vi "ge_CfgGroup.vi"(6 "Group Specific Info":T5={"Rate Class"=enum."Low Speed", "Chassis Name"="cDAQ9188-1630874-007"}, 7 "Mode":enum16{"Cfg", "Run"}(ring), 8 "error in":errorcluster, 11 "ChanGrp.lvclass":refnum<class "ChanGrp.lvclass">) -> (0 "error out":errorcluster, 2 "Canceled?":bool, 3 "ChanGrp.lvclass":refnum<class "ChanGrp.lvclass">)   [LabVIEW 2018]
uses:
  Custom Ctls Table/ge_PullDown.ctl
  Custom Buttons/Reset_Blue.ctl
  Classes/Cfg Grandmaster/Class Chan Group/ChanGrp.lvclass
  Custom Ctls Table/ge_CellInt.ctl
  Custom Ctls Table/ge_GrpSpecificInfo.ctl
  Common/Controls/TE_Designator.ctl
  Custom Ctls Table/ge_CellString.ctl
  Custom Ctls Table/ge_CellHiLite.ctl
  Custom Buttons/Open_BlueSmall.ctl
  Custom Buttons/Save_BlueSmall.ctl
  <vilib>/event_ctls.llb/eventvkey.ctl
  Custom Ctls Table/ge_TableCmnds.ctl
  Custom Ctls Table/ge_CellContents.ctl
  <vilib>/Utility/miscctls.llb/LVPoint32TypeDef.ctl
  <vilib>/Utility/inputDevices.llb/mouseAcquire.vi
  <vilib>/Utility/inputDevices.llb/closeMouse.vi
panel:
  in  "Save Channel List":T1
  in  "Load Descriptions":T2
  in  "Cal2":bool
  in  "Bool1":bool
  in  "CellHiLite":T3
  in  "CellString":T4=" Quarter Bridge I"
  in  "Cal1":bool
  in  "Cal0":bool
  in  "Dbl6":dbl
  in  "Dbl5":dbl=1000.0
  in  "Dbl4":dbl=1000.0
  in  "Dbl3":dbl=1000.0
  in  "Dbl2":dbl
  in  "Dbl1":dbl=1.0
  in  "Ring3":u16(ring)=10050 items=["RMS"=1, "Peak"=0, ""=65535]
  in  "CellInt":T7
  in  "CellDbl":dbl
  in  "Bool0":bool
  in  "Int0":i32
  in  "Str0":string="V"
  in  "Dbl0":dbl=25.0 format="%#.6g"
  in  "Cancel":bool
  in  "Reset":T8
  in  "Ring2":u16(ring)=10200 items=["Full Bridge I"=10183, "Full Bridge II"=10184, "Full Bridge III"=10185, "Half Bridge I"=10188, "Half Bridge II"=10189, "Quarter Bridge I"=10271, "Quarter Bridge II"=10272, ""=65535]
  in  "Ring1":u16(ring)=10086 items=["10 V"=10000, "5 V"=5000, "3.3 V"=3300, "2.5 V"=2500, ""=65535]
  in  "Ring0":u16(ring)=10144 items=["High Res"=0, ""=65535]
  in  "Pull Down":T9=65535 items=["Quarter Bridge II"=10272, "Quarter Bridge I"=10271, "Half Bridge II"=10189, "Half Bridge I"=10188, "Full Bridge III"=10185, "Full Bridge II"=10184, "Full Bridge I"=10183, ""=65535]
  in  "Apply":bool
  in  "Chan Table":i32[](listbox)
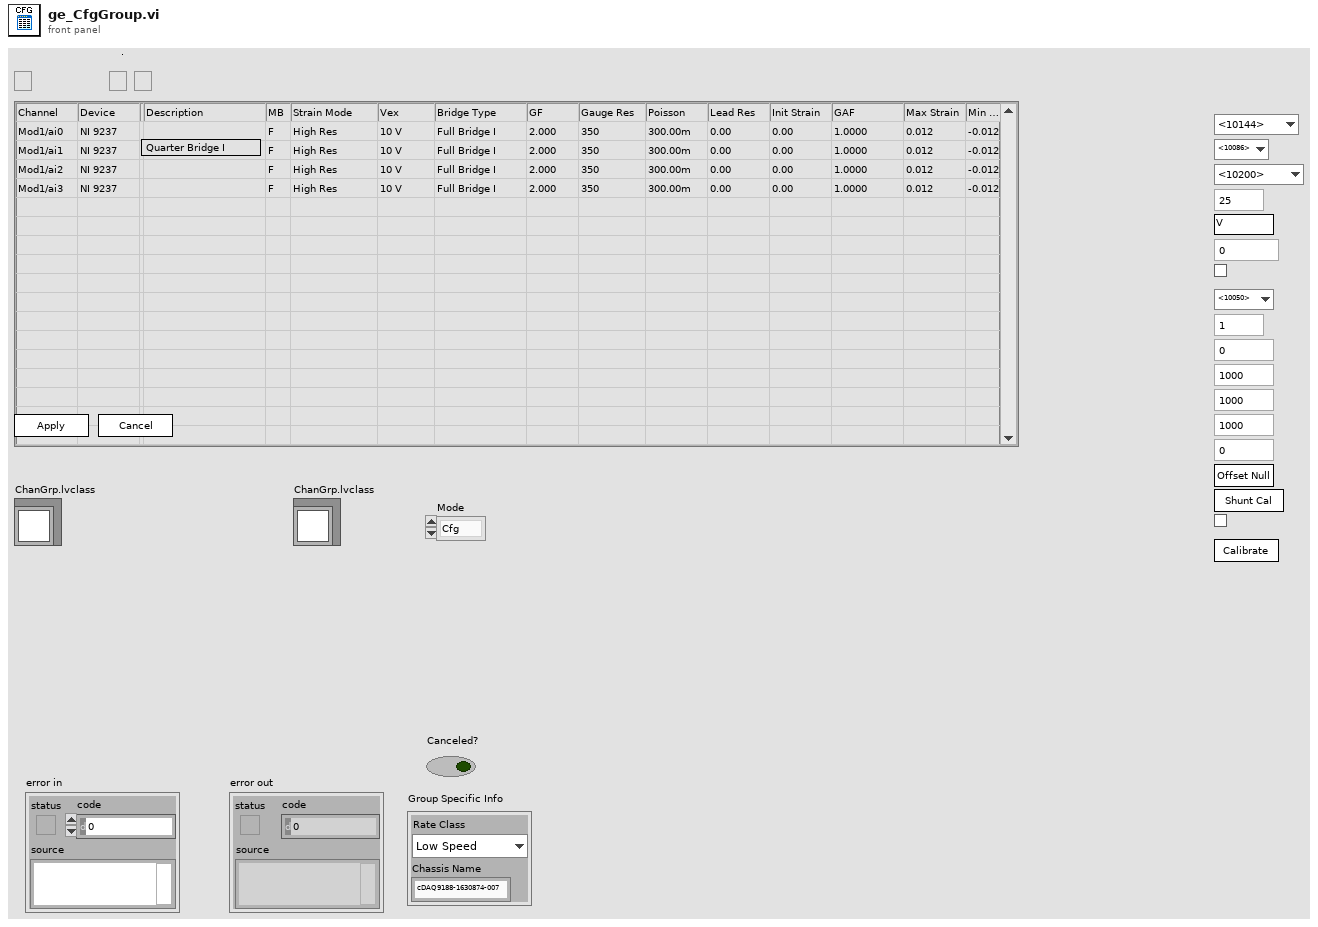
[diagram p1: front panel]
types:
  T1 = typedef "Save_BlueSmall.ctl" = bool
  T2 = typedef "Open_BlueSmall.ctl" = bool
  T3 = typedef "ge_CellHiLite.ctl" = bool
  T4 = typedef "ge_CellString.ctl" = string
  T5 = typedef "ge_GrpSpecificInfo.ctl" = cluster{"Rate Class":T6, "Chassis Name":string}
  T6 = typedef "TE_Designator.ctl" = enum16{"High Speed", "Low Speed"}
  T7 = typedef "ge_CellInt.ctl" = i32
  T8 = typedef "Reset_Blue.ctl" = bool
  T9 = typedef "ge_PullDown.ctl" = u16
  T10 = typedef "eventvkey.ctl" = enum16{"ASCII", "Enter", "Return", "Shift", "Ctrl", "Alt", "Cmd", "Opt", "Caps", "NumLock", "Clear", "Break", "Up", "Down", "Left", "Right", "Insert", "Delete", "Home", "End", "PageUp", "PageDown", "Escape", "Help", "Pause", "ScrollLock", "F1", "F2", "F3", "F4", "F5", "F6", "F7", "F8", "F9", "F10", "F11", "F12", "F13", "F14", "F15", "F16", "F17", "F18", "F19", "F20", "F21", "F22", "F23", "F24", "Play", "VolumeUp", "VolumeDown", "Mute", "Two Byte Char"}
  T11 = typedef "ge_TableCmnds.ctl" = enum16{"Initialize", "Hide Cell Ctrls", "Position Ctrls", "Load Table", "Reset Table", "Clear Selections", "Ungchd Enter?", "Cell ValChng", "Click Ring", "Edit Cell", "Dismiss Menu", "Glbl Apply", "Calibrate", "Apply Settings", "Cell Key", "SaveChanList", "LoadChanDesc", "Shutdown"}
  T12 = enum32{"Invalid", "Standard", "Closed", "Hidden", "Minimized", "Maximized"}
  T13 = cluster{"This VI":refnum<vi>, "Group Specific Info":T5}
  T14 = typedef "ge_CellContents.ctl" = cluster{"Cell Contents":cluster{"Cell Text":string, "Cell BG Color":u32}, "Coords":T15}
  T15 = typedef "LVPoint32TypeDef.ctl" = cluster{"Horizontal":i32, "Vertical":i32}
  T16 = cluster{"Horizontal":i32, "Vertical":i32, "Scrolling":i32}
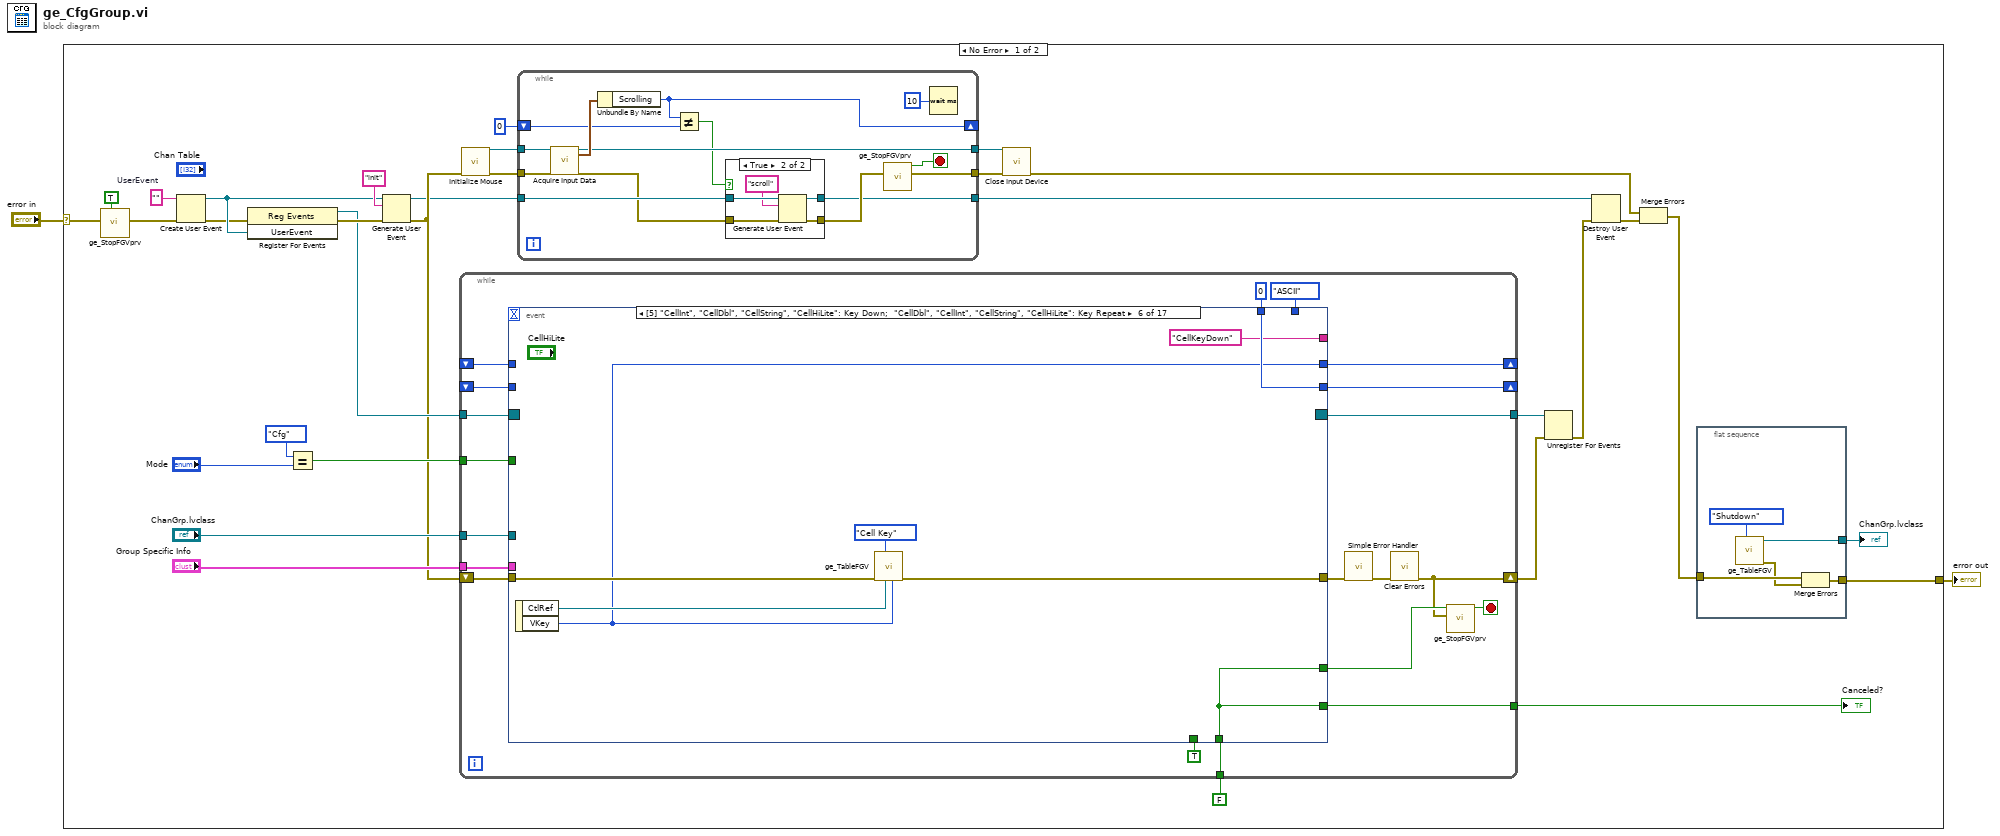
[diagram p0: block diagram]
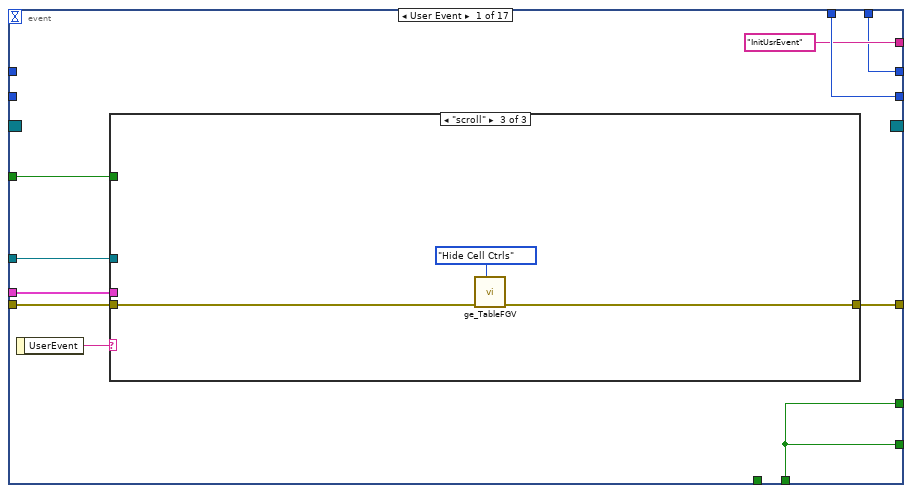
[diagram p3: hidden frame]
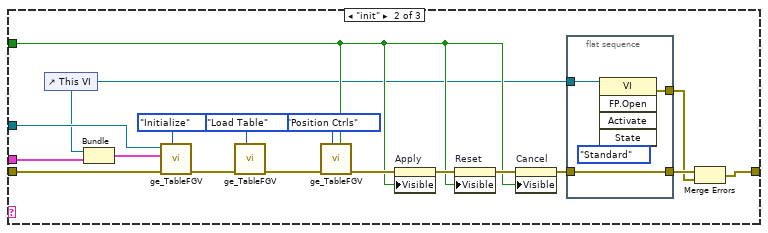
[diagram p5: hidden frame]
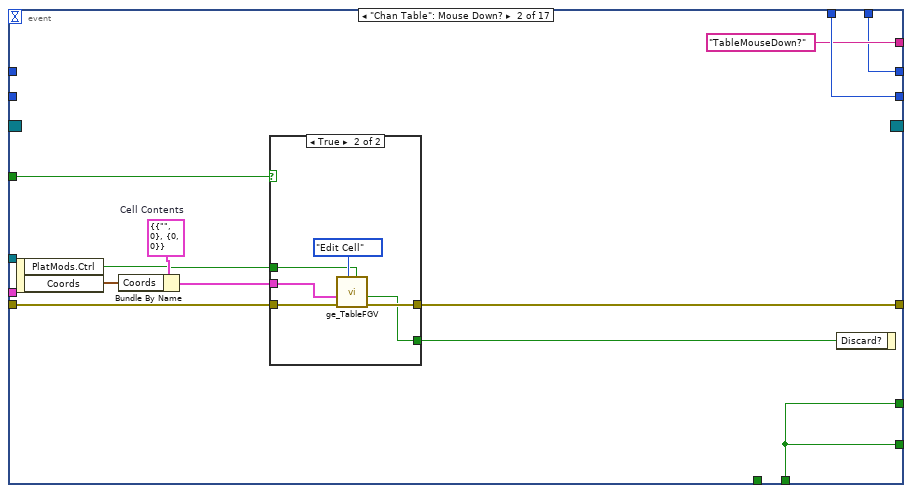
[diagram p6: hidden frame]
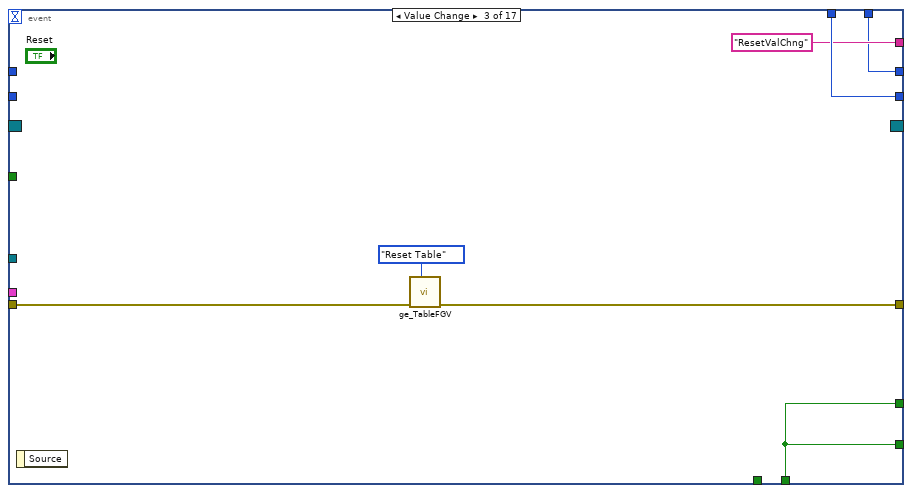
[diagram p8: hidden frame]
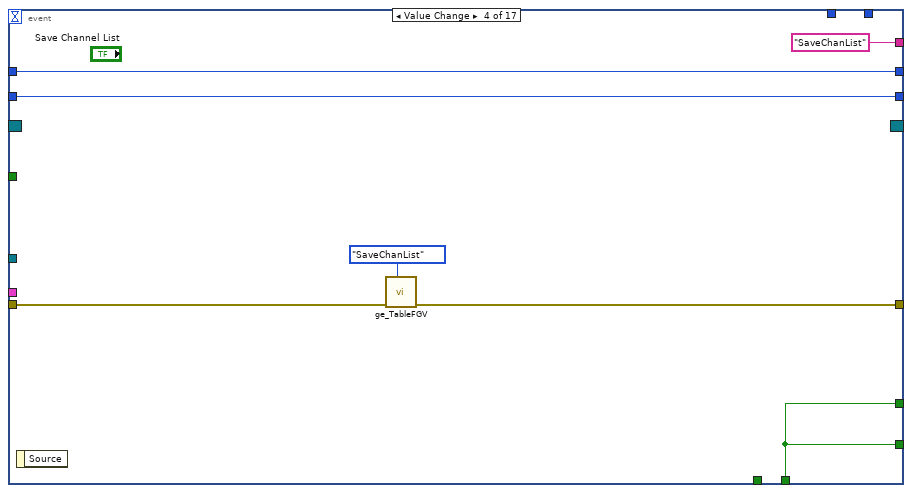
[diagram p9: hidden frame]
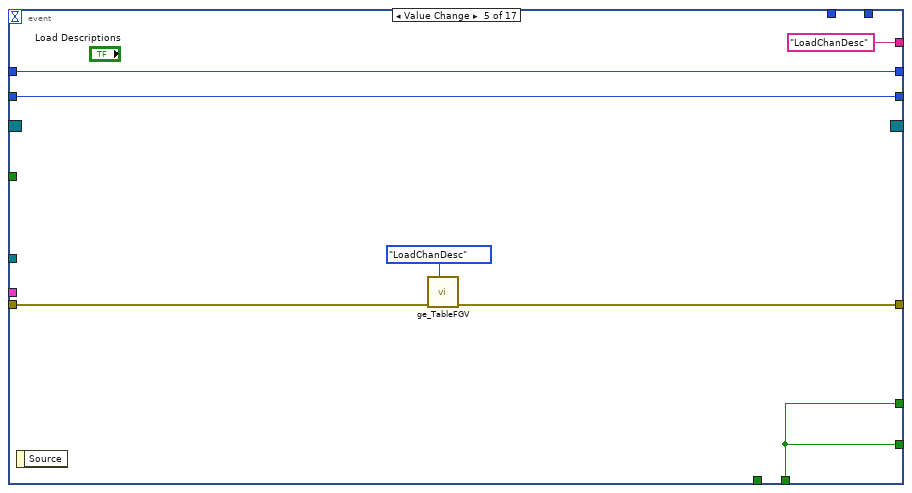
[diagram p10: hidden frame]
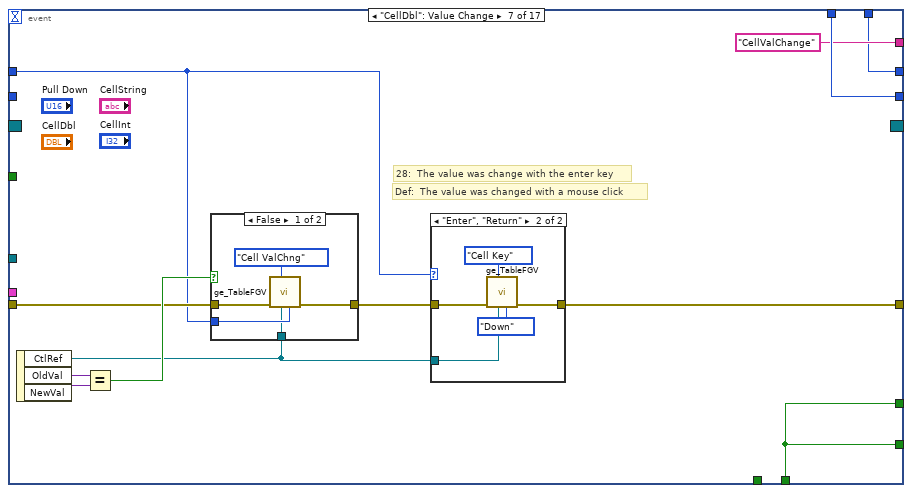
[diagram p11: hidden frame]
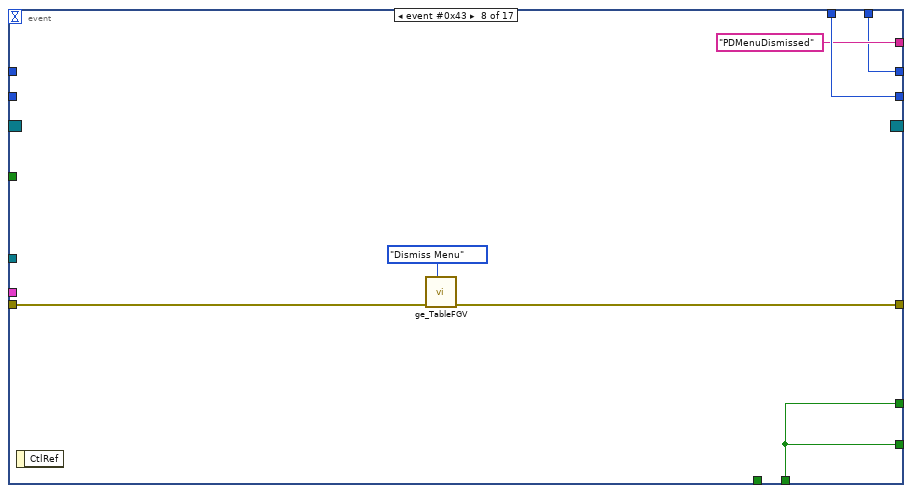
[diagram p14: hidden frame]
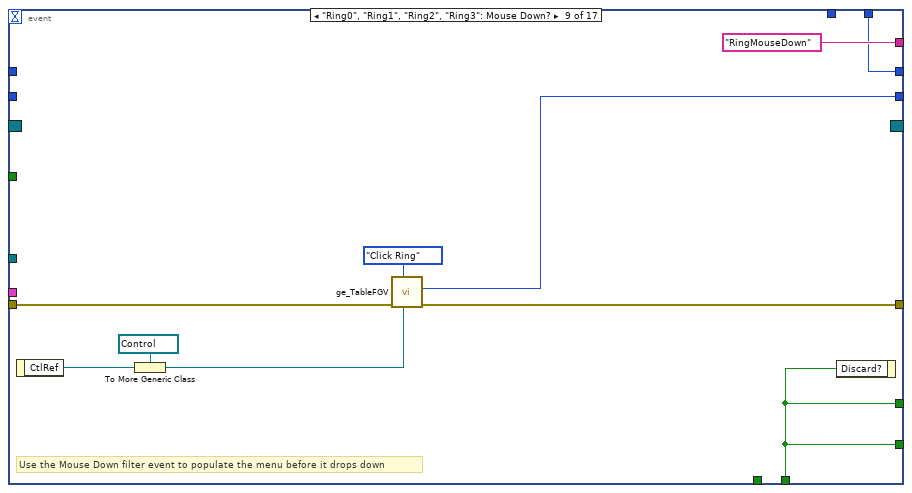
[diagram p15: hidden frame]
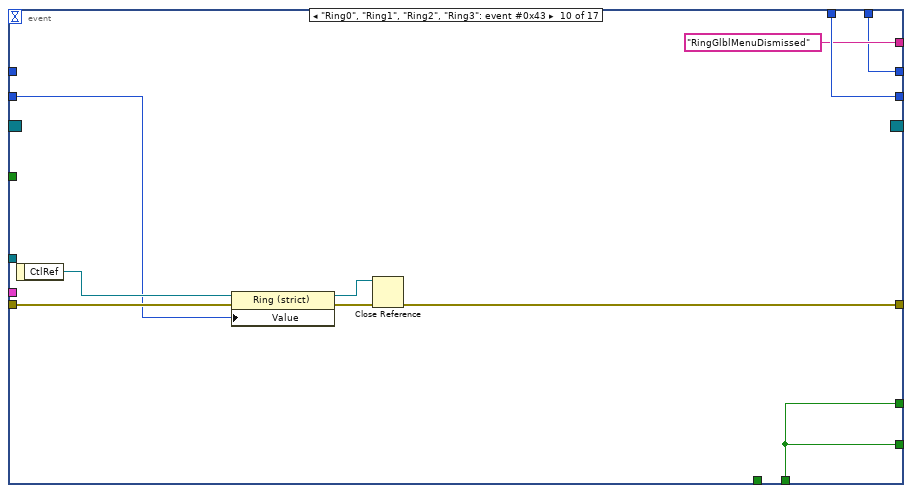
[diagram p16: hidden frame]
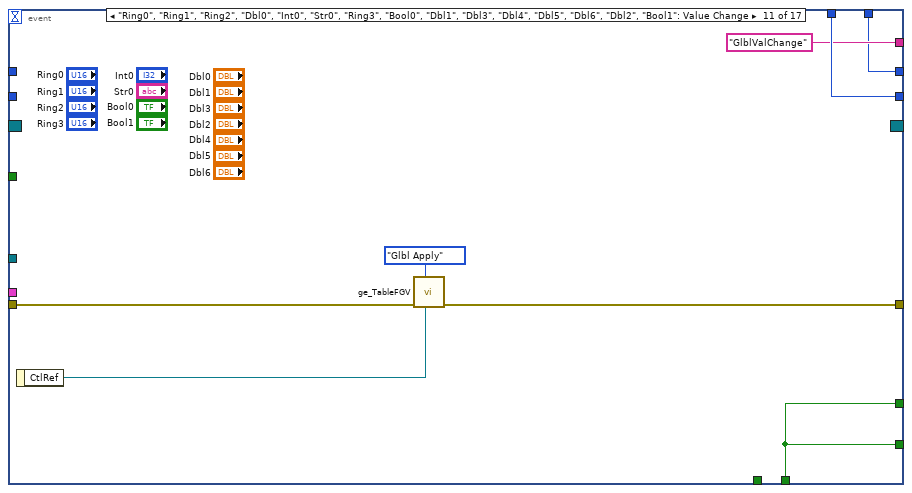
[diagram p17: hidden frame]
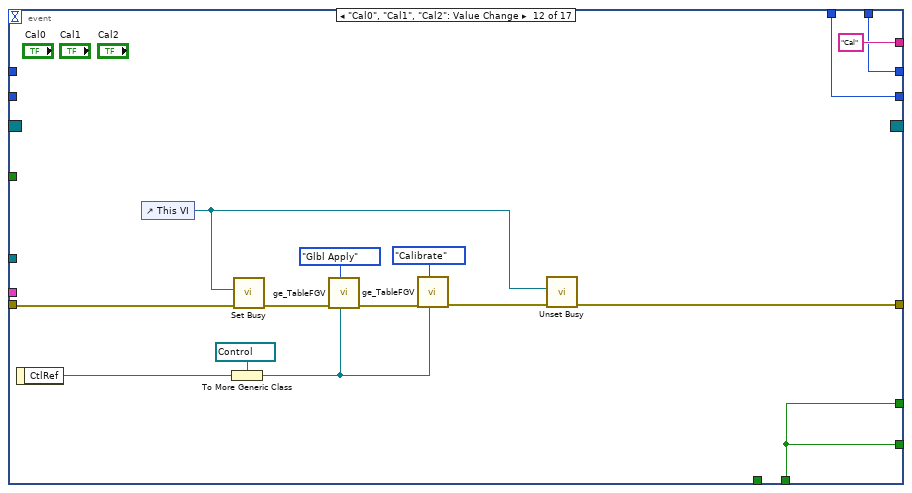
[diagram p18: hidden frame]
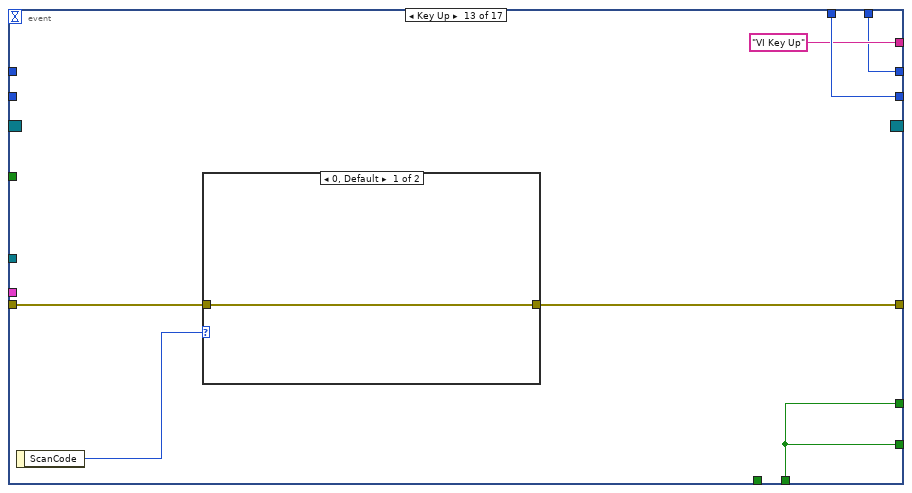
[diagram p19: hidden frame]
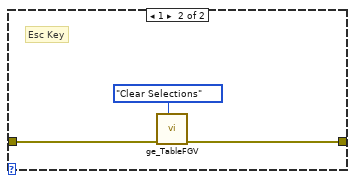
[diagram p20: hidden frame]
diagram:
  n1 = case shown="No Error" "error in" {
    selector: "error in" -> [w7 w284]
    tunnel: [w34 w284] -> w1
    frame No Error {
      w31 = ""  # UserEvent
      n2 = call "ge_StopFGVprv.vi"("Reset (F)"=TRUE, "error in"=w7) -> ("error out"=w6:errorcluster)  [unwired: 8 in, 1 out]
      n3 = Create User Event(user event datatype=w31, error in=w6) -> (user event=w29:refnum<user-event>, error out=w28:errorcluster)
      n4 = register-events(error in=w28, w29) -> (reference out=w27:refnum<event-registration>, error out=w30:errorcluster)  [unwired: 1 in]
      n5 = Equal?(x=enum16{"Cfg", "Run"}."Cfg", y="Mode") -> (x = y?=w19:bool)
      n6 = Generate User Event(user event=w29, event data cluster="init" ("event data"), error in=w30) -> (user event out=w4:refnum<user-event>, error out=w13:errorcluster)  [unwired: 1 in]
      n7 = while {
        shift-right: [w56] -> w24
        shift-left: w13 -> [w75]
        tunnel: w19 -> [w74]
        tunnel: [w72] -> w22
        tunnel: FALSE ("Apply") -> [w67]
        tunnel: "ChanGrp.lvclass" -> [w71]
        tunnel: w27 -> [w70]
        tunnel: [w69] -> w25
        shift-right: [w68] -> _
        shift-left: _ -> [w66]
        tunnel: "Group Specific Info" -> [w65]
        shift-right: [w62] -> _
        shift-left: _ -> [w61]
        stop <- w58 stop-if-true
        n8 = event shown="[5] \"CellInt\", \"CellDbl\", \"CellString\", \"CellHiLite\": Key Down;  \"CellDbl\", \"CellInt\", \"CellString\", \"CellHiLite\": Key Repeat" {
          selector: w70 -> [_ _ _ _ _ _ _ _ _ _ _ _ _ _ _ _ _]
          dyn-events: [_ _ _ _ _ _ _ _ _ _ _ _ _ _ _ _ _] -> w69
          timeout: _ -> [_ _ _ _ _ _ _ _ _ _ _ _ _ _ _ _ _]
          tunnel: [w84 w121 w135 w142 w149 w160 w172 w188 w192 w207 w219 w234 w239 w252 w265 w272 w277] -> w57
          tunnel: [w77 w123 w137 w139 w146 w158 w171 w190 w198 w208 w217 w226 w241 w250 w267 w273 w278] -> w64
          tunnel: w75 -> [w85 w122 w138 w140 w147 w159 w166 w189 w200 w210 w216 w229 w240 w253 w268 w273 w278]
          tunnel: w74 -> [w81 w115 _ _ _ _ _ _ _ _ _ _ _ _ _ _ _]
          tunnel: TRUE -> [_ _ _ _ _ _ _ _ _ _ _ _ _ _ w265 w272 w277]
          tunnel: [w84 w121 w135 w142 w149 w160 w172 w188 w192 w207 w219 w234 w239 w252 w264 w272 w277] -> w72
          tunnel: w71 -> [w83 _ _ _ _ _ _ _ _ _ _ _ _ _ _ _ _]
          tunnel: [w78 w112 w132 w144 w152 w153 w162 w185 w193 w204 w212 w220 w235 w246 w261 w269 w274] -> w68
          tunnel: w67 -> [w84 w121 w135 w142 w149 w160 w172 w188 w192 w207 w219 w234 w239 w252 w264 _ _]
          tunnel: w66 -> [_ _ _ w144 w152 _ w164 _ _ _ _ _ _ _ _ _ _]
          tunnel: w65 -> [w82 _ _ _ _ _ _ _ _ _ _ _ _ _ _ _ _]
          tunnel: [w80 w114 w134 w143 w151 w157 w165 w187 w199 w206 w214 w230 w237 w248 w263 w271 w276] -> w62
          tunnel: w61 -> [_ _ _ w143 w151 _ _ _ _ w202 _ _ _ _ _ _ _]
          tunnel: u16 0 ("RingVal") -> [w80 w114 w134 _ _ w157 w165 w187 _ w206 w214 w230 w237 w248 w263 w271 w276]
          tunnel: ["InitUsrEvent" "TableMouseDown?" "ResetValChng" "SaveChanList" "LoadChanDesc" "CellKeyDown" "CellValChange" "PDMenuDismissed" "RingMouseDown" "RingGlblMenuDismissed" "GlblValChange" "Cal" "VI Key Up" "PaneMouseDn" "ApplyValChng" "CancelValChng" "PanelClose?"] -> _
          tunnel: eventvkey."ASCII" ("VKey") -> [w78 w112 w132 _ _ _ w162 w185 w193 w204 w212 w220 w235 w246 w261 w269 w274]
          event User Event {
            n9 = event-data() -> ("UserEvent"=w76:string)  [unwired: 1 in]
            n10 = case shown="\"scroll\"" w76 {
              tunnel: w85 -> [w86 w103 w110]
              tunnel: w83 -> [_ w102 _]
              tunnel: w82 -> [_ w94 _]
              tunnel: w81 -> [_ w92 _]
              tunnel: [w86 w87 w109] -> w77
              frame Default {
              }
              frame "init" {
                n11 = control-ref of="This VI"() -> (w91:refnum<vi>)
                n12 = Bundle("This VI"=w91, "Group Specific Info"=w94) -> (w93:T13)  [unwired: 1 in]
                n13 = call "ge_TableFGV.vi"("ge_TableCmnds"=ge_TableCmnds."Initialize" ("ge_VoltTableCmnds"), "error in"=w103, "Specific Info"=w93, "ChanGrp.lvclass"=w102) -> ("error out"=w98:errorcluster)  [unwired: 4 in, 3 out]
                n14 = call "ge_TableFGV.vi"("ge_TableCmnds"=ge_TableCmnds."Load Table" ("ge_VoltTableCmnds"), "error in"=w98) -> ("error out"=w96:errorcluster)  [unwired: 6 in, 3 out]
                n15 = call "ge_TableFGV.vi"("Mod"=w92, "ge_TableCmnds"=ge_TableCmnds."Position Ctrls" ("ge_VoltTableCmnds"), "error in"=w96) -> ("error out"=w95:errorcluster)  [unwired: 5 in, 3 out]
                n16 = property on="Apply" class="Bool"(error in=w95, "Visible"=w92) -> (error out=w101:errorcluster)  [unwired: 1 in, 1 out]
                n17 = property on="Reset" class="Bool"(error in=w101, "Visible"=w92) -> (error out=w100:errorcluster)  [unwired: 1 in, 1 out]
                n18 = property on="Cancel" class="Bool"(error in=w100, "Visible"=w92) -> (error out=w90:errorcluster)  [unwired: 1 in, 1 out]
                n19 = flat-sequence {
                  tunnel: [w108] -> w88
                  tunnel: w91 -> [w106]
                  tunnel: w90 -> [w105]
                  tunnel: [w105] -> w89
                  frame #0 {
                    n20 = invoke class="VI" method="FP.Open"(reference=w106, "State"=T12."Standard") -> (error out=w108:errorcluster)  [unwired: 3 in, 4 out]
                  }
                }
                n21 = Merge Errors(w89, w88) -> (w87:errorcluster)
              }
              frame "scroll" {
                n22 = call "ge_TableFGV.vi"("ge_TableCmnds"=ge_TableCmnds."Hide Cell Ctrls" ("ge_VoltTableCmnds"), "error in"=w110) -> ("error out"=w109:errorcluster)  [unwired: 6 in, 3 out]
              }
            }
          }
          event "Chan Table": Mouse Down? {
            w120 = T14 {"Cell Contents"={"Cell Text"="", "Cell BG Color"=0}, "Coords"={"Horizontal"=0, "Vertical"=0}}  # Cell Contents
            n23 = event-data() -> ("PlatMods.Ctrl"=w116:bool, "Coords"=w119:T15)  [unwired: 1 in]
            n24 = Bundle By Name(cluster=w120, "Coords"=w119) -> (w118:T14)
            n25 = case shown="True" w115 {
              selector: w115 -> [w124 _]
              tunnel: [w125 w131] -> w123
              tunnel: w122 -> [w125 w130]
              tunnel: w118 -> [_ w128]
              tunnel: [w124 w126] -> w117
              tunnel: w116 -> [_ w127]
              frame False {
              }
              frame True {
                n26 = call "ge_TableFGV.vi"("Mod"=w127, "ge_TableCmnds"=ge_TableCmnds."Edit Cell" ("ge_VoltTableCmnds"), "error in"=w130, "Cell Contents"=w128) -> ("error out"=w131:errorcluster, "Discard?"=w126:bool)  [unwired: 4 in, 2 out]
              }
            }
            n27 = event-data("Discard?"=w117) -> ()  [unwired: 1 in, 1 out]
          }
          event Value Change {
            n28 = event-data() -> ()  [unwired: 1 in, 1 out]
            n29 = call "ge_TableFGV.vi"("ge_TableCmnds"=ge_TableCmnds."Reset Table" ("ge_VoltTableCmnds"), "error in"=w138) -> ("error out"=w137:errorcluster)  [unwired: 6 in, 3 out]
          }
          event Value Change {
            n30 = event-data() -> ()  [unwired: 1 in, 1 out]
            n31 = call "ge_TableFGV.vi"("ge_TableCmnds"=ge_TableCmnds."SaveChanList" ("ge_VoltTableCmnds"), "error in"=w140) -> ("error out"=w139:errorcluster)  [unwired: 6 in, 3 out]
          }
          event Value Change {
            n32 = event-data() -> ()  [unwired: 1 in, 1 out]
            n33 = call "ge_TableFGV.vi"("ge_TableCmnds"=ge_TableCmnds."LoadChanDesc" ("ge_VoltTableCmnds"), "error in"=w147) -> ("error out"=w146:errorcluster)  [unwired: 6 in, 3 out]
          }
          event "CellDbl": Key Down; "CellDbl": Key Repeat {
            n34 = event-data() -> ("CtlRef"=w155:refnum<vi>, "VKey"=w153:T10)  [unwired: 1 in]
            n35 = call "ge_TableFGV.vi"("VKey"=w153, "CtlRef"=w155, "ge_TableCmnds"=ge_TableCmnds."Cell Key" ("ge_VoltTableCmnds"), "error in"=w159) -> ("error out"=w158:errorcluster)  [unwired: 4 in, 3 out]
          }
          event "CellDbl": Value Change {
            # "Def:  The value was changed with a mouse click"
            # "28:  The value was change with the enter key"
            n36 = event-data() -> ("CtlRef"=w161:refnum<vi>, "OldVal"=w169:variant, "NewVal"=w167:variant)  [unwired: 1 in]
            n37 = Equal?(x=w169, y=w167) -> (x = y?=w168:bool)
            n38 = case shown="False" w168 {
              tunnel: w166 -> [w177 w178]
              tunnel: [w175 w178] -> w170
              tunnel: w164 -> [w174 _]
              tunnel: w161 -> [w173 _]
              frame False {
                n39 = call "ge_TableFGV.vi"("VKey"=w174, "CtlRef"=w173, "ge_TableCmnds"=ge_TableCmnds."Cell ValChng" ("ge_VoltTableCmnds"), "error in"=w177) -> ("error out"=w175:errorcluster)  [unwired: 4 in, 3 out]
              }
              frame True {
              }
            }
            n40 = case shown="\"Enter\", \"Return\"" w164 {
              tunnel: [w179 w182] -> w171
              tunnel: w170 -> [w179 w183]
              tunnel: w161 -> [_ w180]
              frame Default {
              }
              frame "Enter", "Return" {
                n41 = call "ge_TableFGV.vi"("VKey"=eventvkey."Down", "CtlRef"=w180, "ge_TableCmnds"=ge_TableCmnds."Cell Key" ("ge_VoltTableCmnds"), "error in"=w183) -> ("error out"=w182:errorcluster)  [unwired: 4 in, 3 out]
              }
            }
          }
          event event #0x43 {
            n42 = event-data() -> ()  [unwired: 1 in, 1 out]
            n43 = call "ge_TableFGV.vi"("ge_TableCmnds"=ge_TableCmnds."Dismiss Menu" ("ge_VoltTableCmnds"), "error in"=w189) -> ("error out"=w190:errorcluster)  [unwired: 6 in, 3 out]
          }
          event "Ring0", "Ring1", "Ring2", "Ring3": Mouse Down? {
            # "Use the Mouse Down filter event to populate the menu before it drops down"
            n44 = event-data() -> ("CtlRef"=w196:refnum<vi>)  [unwired: 1 in]
            n45 = To More Generic Class(target class=refnum<vi> refnum ("CtlRef"), reference=w196) -> (generic class reference=w195:refnum<vi>)
            n46 = call "ge_TableFGV.vi"("CtlRef"=w195, "ge_TableCmnds"=ge_TableCmnds."Click Ring" ("ge_VoltTableCmnds"), "error in"=w200) -> ("error out"=w198:errorcluster, "ValIfDismissed"=w199:u16)  [unwired: 5 in, 2 out]
            n47 = event-data("Discard?"=w192) -> ()  [unwired: 1 in, 1 out]
          }
          event "Ring0", "Ring1", "Ring2", "Ring3": event #0x43 {
            n48 = event-data() -> ("CtlRef"=w209:refnum<vi>)  [unwired: 1 in]
            n49 = property on="Property Node" class="Ring (strict)"(reference=w209, error in=w210, "Value"=w202) -> (reference out=w203:refnum<vi>, error out=w211:errorcluster)
            n50 = Close Reference(reference=w203, error in (no error)=w211) -> (error out=w208:errorcluster)
          }
          event "Ring0", "Ring1", "Ring2", "Dbl0", "Int0", "Str0", "Ring3", "Bool0", "Dbl1", "Dbl3", "Dbl4", "Dbl5", "Dbl6", "Dbl2", "Bool1": Value Change {
            n51 = event-data() -> ("CtlRef"=w215:refnum<vi>)  [unwired: 1 in]
            n52 = call "ge_TableFGV.vi"("CtlRef"=w215, "ge_TableCmnds"=ge_TableCmnds."Glbl Apply" ("ge_VoltTableCmnds"), "error in"=w216) -> ("error out"=w217:errorcluster)  [unwired: 5 in, 3 out]
          }
          event "Cal0", "Cal1", "Cal2": Value Change {
            n53 = event-data() -> ("CtlRef"=w224:refnum<vi>)  [unwired: 1 in]
            n54 = control-ref of="This VI"() -> (w225:refnum<vi>)
            n55 = To More Generic Class(target class=refnum<vi> refnum ("CtlRef"), reference=w224) -> (generic class reference=w222:refnum<vi>)
            n56 = call <vilib>:"Set Busy.vi"("error in (no error)"=w229, "VI reference (current VI)"=w225) -> ("error out"=w228:errorcluster)  [unwired: 8 in, 1 out]
            n57 = call "ge_TableFGV.vi"("CtlRef"=w222, "ge_TableCmnds"=ge_TableCmnds."Glbl Apply" ("ge_VoltTableCmnds"), "error in"=w228) -> ("error out"=w231:errorcluster)  [unwired: 5 in, 3 out]
            n58 = call "ge_TableFGV.vi"("CtlRef"=w222, "ge_TableCmnds"=ge_TableCmnds."Calibrate" ("ge_VoltTableCmnds"), "error in"=w231) -> ("error out"=w227:errorcluster)  [unwired: 5 in, 3 out]
            n59 = call <vilib>:"Unset Busy.vi"("error in (no error)"=w227, "VI reference (current VI)"=w225) -> ("error out"=w226:errorcluster)  [unwired: 9 in]
          }
          event Key Up {
            n60 = event-data() -> ("ScanCode"=w238:i16)  [unwired: 1 in]
            n61 = case shown="0, Default" w238 {
              tunnel: [w242 w243] -> w241
              tunnel: w240 -> [w242 w244]
              frame 0, Default {
              }
              frame 1 {
                # "Esc Key"
                n62 = call "ge_TableFGV.vi"("ge_TableCmnds"=ge_TableCmnds."Clear Selections" ("ge_VoltTableCmnds"), "error in"=w244) -> ("error out"=w243:errorcluster)  [unwired: 6 in, 3 out]
              }
            }
          }
          event Mouse Down? {
            # "Right Click"
            n63 = event-data() -> ("Button"=w256:u16)  [unwired: 1 in]
            n64 = Equal?(x=u16 2, y=w256) -> (x = y?=w254:bool)
            n65 = case shown="True" w254 {
              tunnel: [w257 w259] -> w251
              tunnel: w253 -> [w257 w260]
              frame False {
              }
              frame True {
                n66 = call "ge_TableFGV.vi"("ge_TableCmnds"=ge_TableCmnds."Clear Selections" ("ge_VoltTableCmnds"), "error in"=w260) -> ("error out"=w259:errorcluster)  [unwired: 6 in, 3 out]
              }
            }
            n67 = call "ge_TableFGV.vi"("ge_TableCmnds"=ge_TableCmnds."Hide Cell Ctrls" ("ge_VoltTableCmnds"), "error in"=w251) -> ("error out"=w250:errorcluster)  [unwired: 6 in, 3 out]
            n68 = event-data("Discard?"=w254) -> ()  [unwired: 1 in, 1 out]
          }
          event "Apply": Value Change {
            n69 = event-data() -> ()  [unwired: 1 in, 1 out]
            n70 = call "ge_TableFGV.vi"("ge_TableCmnds"=ge_TableCmnds."Apply Settings" ("ge_VoltTableCmnds"), "error in"=w268) -> ("error out"=w267:errorcluster)  [unwired: 6 in, 3 out]
          }
          event "Cancel": Value Change {
            n71 = event-data() -> ()  [unwired: 1 in, 1 out]
          }
          event Panel Close? {
            n72 = event-data() -> ()  [unwired: 1 in, 1 out]
            n73 = event-data("Discard?"=w277) -> ()  [unwired: 1 in, 1 out]
          }
        }
        n74 = call <vilib>:"Simple Error Handler.vi"("error in (no error)"=w64) -> ("error out"=w63:errorcluster)  [unwired: 4 in, 4 out]
        n75 = call <vilib>:"Clear Errors.vi"("error in (no error)"=w63) -> ("error out"=w56:errorcluster)  [unwired: 5 in, 1 out]
        n76 = call "ge_StopFGVprv.vi"("error in"=w56, "User stop? (F)"=w57) -> ("Stop?"=w58:bool)  [unwired: 8 in, 1 out]
      }
      "Canceled?" <- w22
      n77 = call <vilib>:"Initialize Mouse.vi"("error in (no error)"=w13) -> ("error out"=w14:errorcluster, "device ID"=w15:refnum<k1>)  [unwired: 9 in]
      n78 = while {
        shift-right: [w47] -> _
        shift-left: 0 ("Scrolling") -> [w46]
        tunnel: w15 -> [w45]
        tunnel: w14 -> [w44]
        tunnel: [w43] -> w11
        tunnel: [w42] -> w12
        tunnel: w4 -> [w40]
        tunnel: [w36] -> w3
        stop <- w41 stop-if-true
        n79 = call-poly <vilib>:"Acquire Input Data.vi"("device ID"=w45, "error in (no error)"=w44) -> ("device ID"=w43:refnum<k1>, "axis info"=w48:T16, "error out"=w39:errorcluster)  [unwired: 14 in, 1 out]
        n80 = Unbundle By Name(w48) -> ("Scrolling"=w47:i32)
        n81 = Not Equal?(x=w47, y=w46) -> (x != y?=w37:bool)
        n82 = case shown="True" w37 {
          tunnel: w40 -> [w49 w55]
          tunnel: w39 -> [w50 w54]
          tunnel: [w50 w53] -> w38
          tunnel: [w49 w51] -> w36
          frame False {
          }
          frame True {
            n83 = Generate User Event(user event=w55, event data cluster="scroll", error in=w54) -> (user event out=w51:refnum<user-event>, error out=w53:errorcluster)  [unwired: 1 in]
          }
        }
        n84 = call "ge_StopFGVprv.vi"("error in"=w38) -> ("error out"=w42:errorcluster, "Stop?"=w41:bool)  [unwired: 9 in]
        n85 = Wait (ms)(milliseconds to wait=u32 10) -> ()  [unwired: 1 out]
      }
      n86 = call-poly <vilib>:"Close Input Device.vi"("error in (no error)"=w12, "device ID"=w11) -> ("error out"=w10:errorcluster)  [unwired: 8 in]
      n87 = Unregister For Events(event registration refnum=w25, error in=w24) -> (error out=w26:errorcluster)
      n88 = Destroy User Event(user event=w3, error in=w26) -> (error out=w9:errorcluster)
      n89 = Merge Errors(w10, w9) -> (w8:errorcluster)
      n90 = flat-sequence {
        tunnel: w8 -> [w282]
        tunnel: [w281] -> w34
        tunnel: [w279] -> w21
        frame #0 {
          n91 = call "ge_TableFGV.vi"("ge_TableCmnds"=ge_TableCmnds."Shutdown" ("ge_VoltTableCmnds")) -> ("error out"=w280:errorcluster, "ChanGrp.lvclass"=w279:refnum<class "ChanGrp.lvclass">)  [unwired: 7 in, 2 out]
          n92 = Merge Errors(w282, w280) -> (w281:errorcluster)
        }
      }
      "ChanGrp.lvclass" <- w21
    }
    frame Error {
    }
  }
  "error out" <- w1
